vi "SwerveKinematics.vi"(8 "Rotation Center Choice":T1(ring), 9 "Joystick Rotation":dbl(slide) scale=1.0..-1.0, 10 "Joystick Y":dbl(slide) scale=-1.0..1.0, 11 "Joystick X":dbl(slide) scale=1.0..-1.0) -> (0 "Module 3 Velocity (ul)":dbl(slide) scale=0.0..1.0 scale format="%.2f", 1 "Module 2 Velocity (ul)":dbl(slide) scale=0.0..1.0 scale format="%.2f", 2 "Module 1 Velocity (ul)":dbl(slide) scale=0.0..1.0 scale format="%.2f", 3 "Module 0 Velocity (ul)":dbl(slide) scale=0.0..1.0 scale format="%.2f", 4 "Module 2 Angle (deg)":dbl(knob) scale=180.0..-180.0 scale format="%#_6f", 5 "Module 1 Angle (deg)":dbl(knob) scale=180.0..-180.0 scale format="%#_6f", 6 "Module 3 Angle (deg)":dbl(knob) scale=180.0..-180.0 scale format="%#_6f", 7 "Module 0 Angle (deg)":dbl(knob) scale=180.0..-180.0 scale format="%#_6f")   [LabVIEW 2019]
doc: "Performs the kinematics for a rectangular four wheel swerve robot with a selectable center of rotation. Swerve module #0 is located in the front right corner and the modules increment in the counter-clockwise direction."
panel:
  out "Angle 3 (deg) Old":dbl
  out "Angle 2 (deg) Old":dbl
  out "Angle 1 (deg) Old":dbl
  out "Velocity 3 (ul) Old":dbl format="%.2f"
  out "Velocity 2 (ul) Old":dbl format="%.2f"
  out "Velocity 1 (ul) Old":dbl format="%.2f"
  out "Velocity 0 (ul) Old":dbl format="%.2f"
  out "Angle 0 (deg) Old":dbl
  out "Velocity 3 (ul)":dbl format="%.2f"
  out "Velocity 2 (ul)":dbl format="%.2f"
  out "Velocity 1 (ul)":dbl format="%.2f"
  out "Velocity 0 (ul)":dbl format="%.2f"
  out "Angle 3 (deg) New":dbl
  out "Angle 2 (deg) New":dbl
  out "Angle 1 (deg) New":dbl
  out "Angle 0 (deg) New":dbl
  in  "Robot Width (in)":dbl=25.0
  in  "Robot Length (in)":dbl=25.0
  # "\"Front\" of Robot"
  # "M1"
  # "M0"
  # "Left Thumbstick"
  # "Right Thumbstick"
  # "X"
  # "Y"
  # "(0,0)"
  # "+CCW"
  # "M2"
  # "M3"
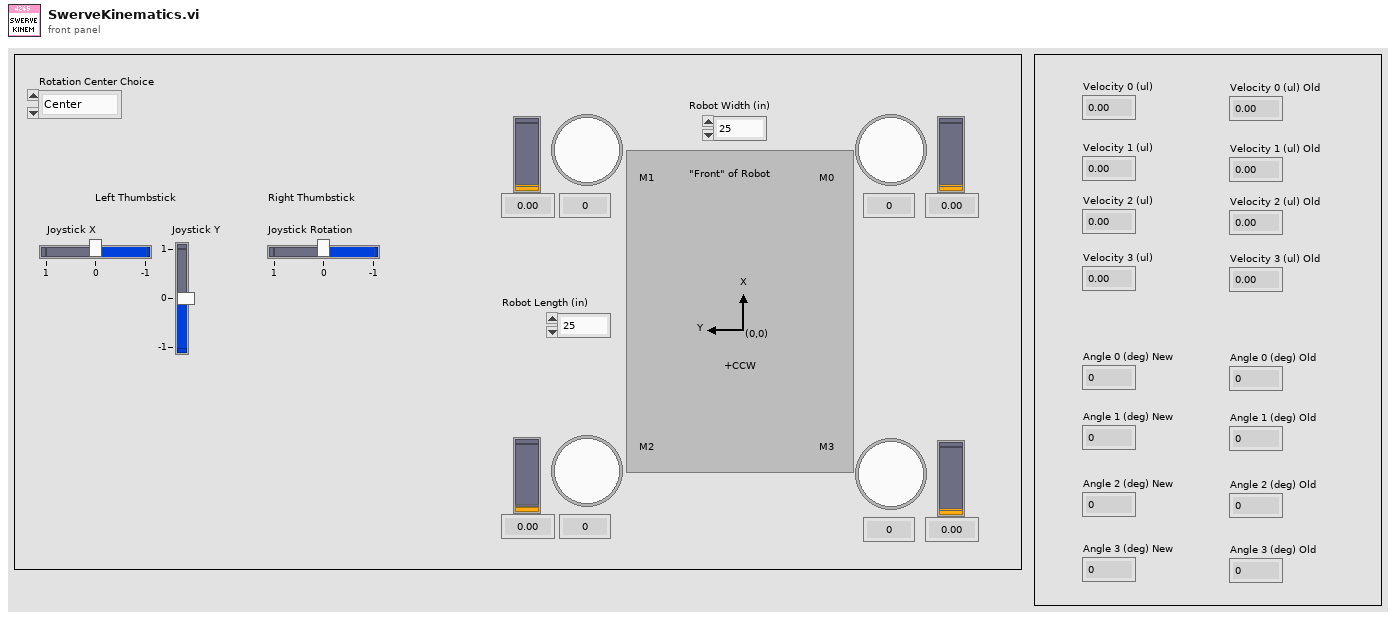
[diagram p1: front panel]
types:
  T1 = enum16{"Center", "Module 0", "Module 1", "Module 2", "Module 3"}
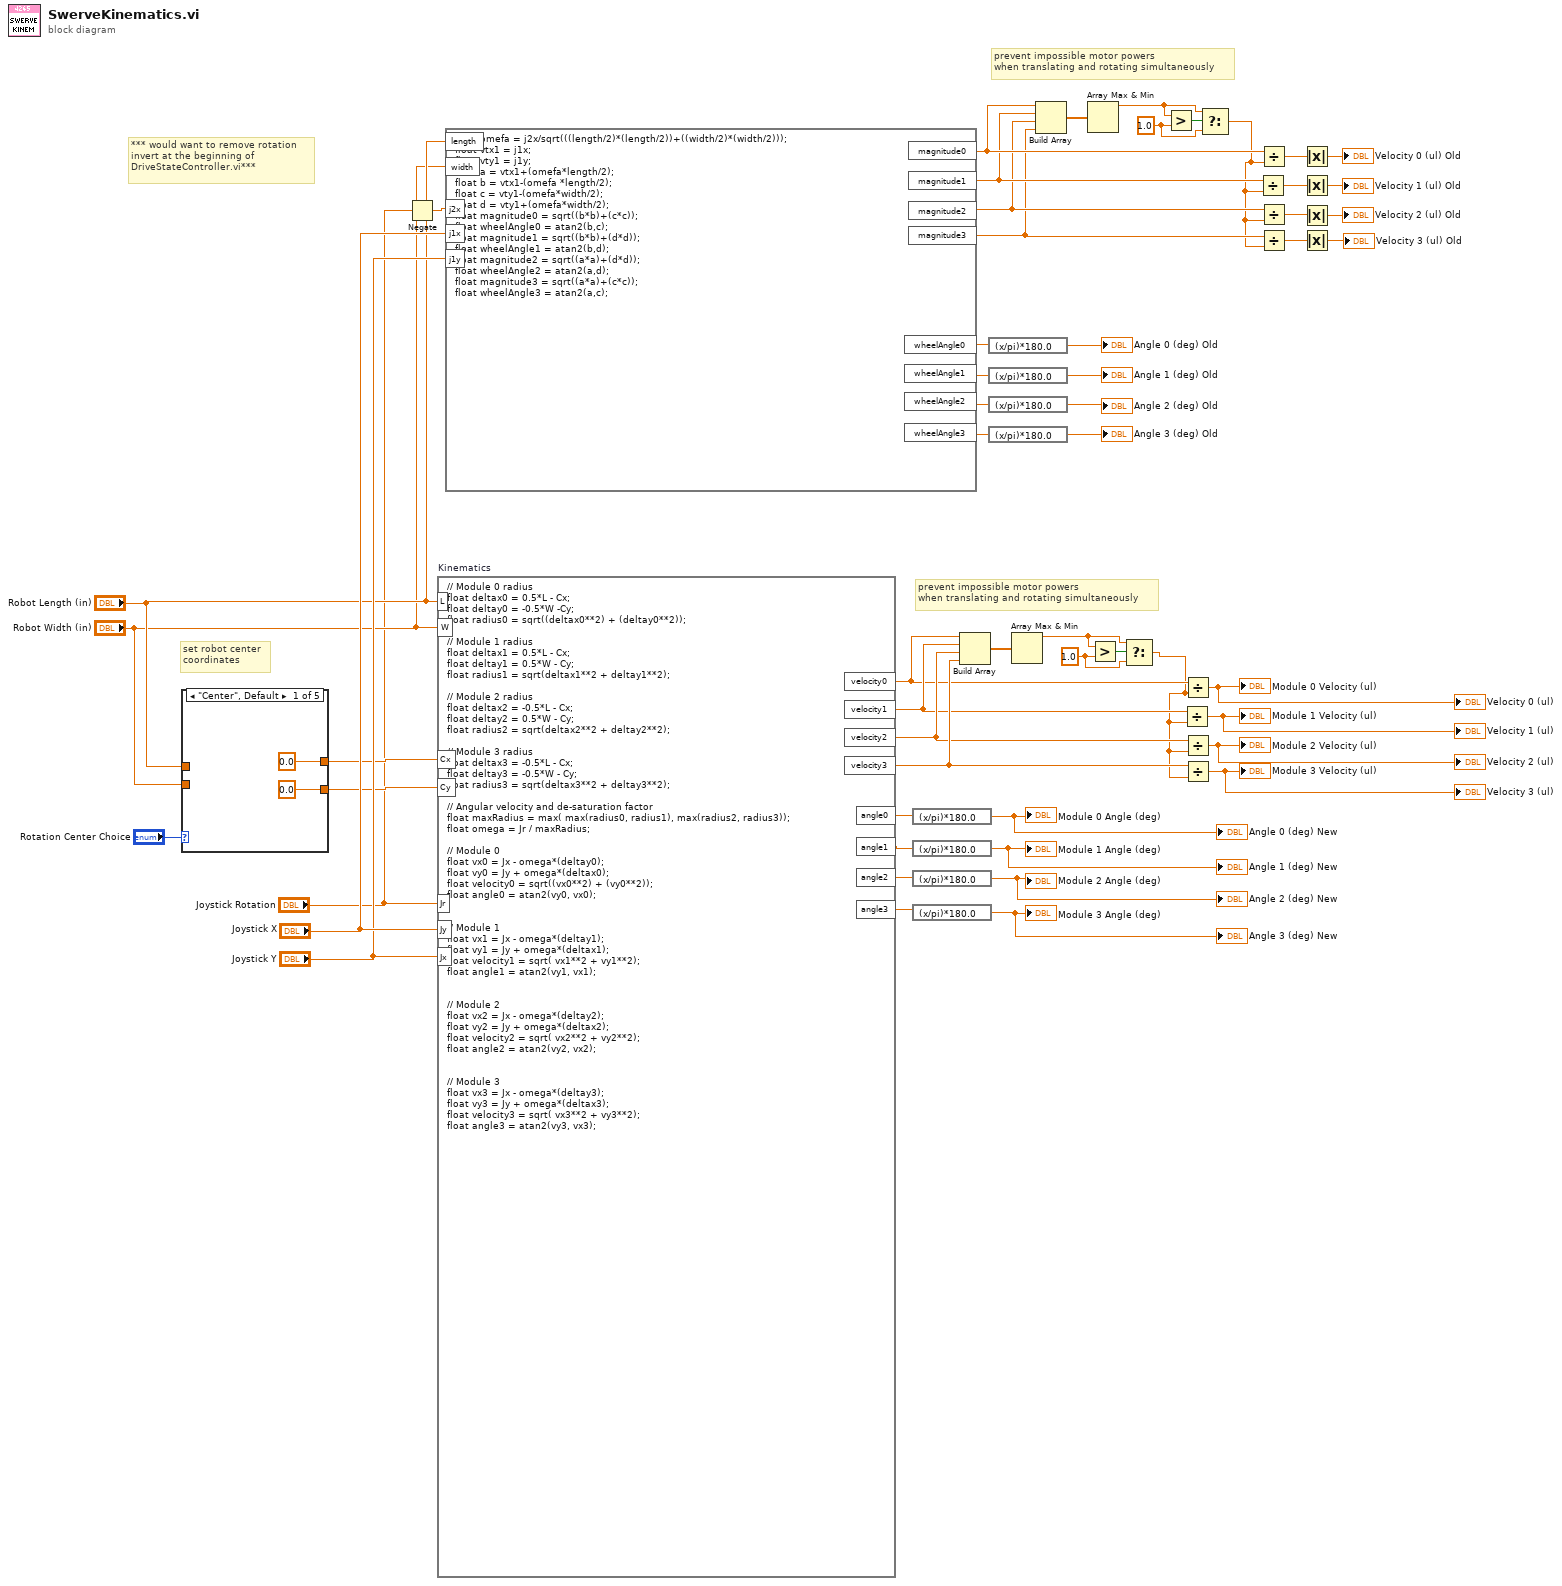
[diagram p0: block diagram]
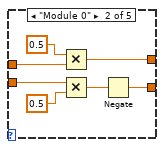
[diagram p2: hidden frame]
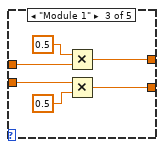
[diagram p3: hidden frame]
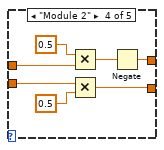
[diagram p4: hidden frame]
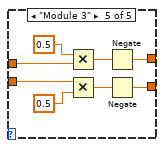
[diagram p5: hidden frame]
diagram:
  w25 = 1.0 ("y")
  w54 = 1.0 ("y")
  # "prevent impossible motor powers\nwhen translating and rotating simultaneously"
  # "set robot center \ncoordinates"
  # "*** would want to remove rotation\ninvert at the beginning of\nDriveStateController.vi***"
  # "prevent impossible motor powers\nwhen translating and rotating simultaneously"
  n1 = case shown="\"Center\", Default" "Rotation Center Choice" {
    tunnel: [0.0 w63 w66 w72 w79] -> w35
    tunnel: [0.0 w58 w65 w71 w78] -> w34
    tunnel: "Robot Length (in)" -> [_ w64 w68 w75 w83]
    tunnel: "Robot Width (in)" -> [_ w61 w67 w74 w82]
    frame "Center", Default {
    }
    frame "Module 0" {
      n2 = Multiply(x=0.5, y=w64) -> (x*y=w63:dbl)
      n3 = Multiply(x=w61, y=0.5) -> (x*y=w60:dbl)
      n4 = Negate(x=w60) -> (-x=w58:dbl)
    }
    frame "Module 1" {
      n5 = Multiply(x=0.5, y=w68) -> (x*y=w66:dbl)
      n6 = Multiply(x=w67, y=0.5) -> (x*y=w65:dbl)
    }
    frame "Module 2" {
      n7 = Multiply(x=0.5, y=w75) -> (x*y=w73:dbl)
      n8 = Multiply(x=w74, y=0.5) -> (x*y=w71:dbl)
      n9 = Negate(x=w73) -> (-x=w72:dbl)
    }
    frame "Module 3" {
      n10 = Multiply(x=0.5, y=w83) -> (x*y=w81:dbl)
      n11 = Multiply(x=w82, y=0.5) -> (x*y=w80:dbl)
      n12 = Negate(x=w81) -> (-x=w79:dbl)
      n13 = Negate(x=w80) -> (-x=w78:dbl)
    }
  }
  n14 = Negate(x="Joystick Rotation") -> (-x=w31:dbl)
  n15 = formula code="// Module 0 radius\nfloat deltax0 = 0.5*L - Cx;\nfloat deltay0 = -0.5*W -Cy; \nfloat radius0 = sqrt((deltax0**2) + (deltay0**2));\n\n// Module 1 radius\nfloat deltax1 = 0.5*L - Cx;\nfloat deltay1 = 0.5*W - Cy;\nfloat radius1 = sqrt(deltax1**2 + deltay1**2);\n\n// Module 2 radius\nfloat deltax2 = -0.5*L - Cx;\nfloat deltay2 = 0.5*W - Cy;\nfloat radius2 = sqrt(deltax2**2 + deltay2**2);\n\n// Module 3 radius\nfloat deltax3 = -0.5*L - Cx;\nfloat deltay3 = -0.5*W - Cy;\nfloat radius3 = sqrt(deltax3**2 + deltay3**2);\n\n// Angular velocity and de-saturation factor\nfloat maxRadius = max( max(radius0, radius1), max(radius2, radius3));\nfloat omega = Jr / maxRadius;\n\n// Module 0\nfloat vx0 = Jx - omega*(deltay0);\nfloat vy0 = Jy + omega*(deltax0);\nfloat velocity0 = sqrt((vx0**2) + (vy0**2));\nfloat angle0 = atan2(vy0, vx0);\n\n\n// Module 1\nfloat vx1 = Jx - omega*(deltay1);\nfloat vy1 = Jy + omega*(deltax1);\nfloat velocity1 = sqrt( vx1**2 + vy1**2);\nfloat angle1 = atan2(vy1, vx1);\n\n\n// Module 2\nfloat vx2 = Jx - omega*(deltay2);\nfloat vy2 = Jy + omega*(deltax2);\nfloat velocity2 = sqrt( vx2**2 + vy2**2);\nfloat angle2 = atan2(vy2, vx2);\n\n\n// Module 3\nfloat vx3 = Jx - omega*(deltay3);\nfloat vy3 = Jy + omega*(deltax3);\nfloat velocity3 = sqrt( vx3**2 + vy3**2);\nfloat angle3 = atan2(vy3, vx3);" "Kinematics"("L"="Robot Length (in)", "W"="Robot Width (in)", "Cx"=w35, "Cy"=w34, "Jr"="Joystick Rotation", "Jx"="Joystick Y", "Jy"="Joystick X") -> ("velocity0"=w19:dbl, "angle0"=w37:dbl, "angle1"=w29:dbl, "angle2"=w28:dbl, "angle3"=w27:dbl, "velocity1"=w20:dbl, "velocity2"=w21:dbl, "velocity3"=w22:dbl)
  n16 = formula code="float omefa = j2x/sqrt(((length/2)*(length/2))+((width/2)*(width/2)));\nfloat vtx1 = j1x;\nfloat vty1 = j1y;\nfloat a = vtx1+(omefa*length/2);\nfloat b = vtx1-(omefa *length/2);\nfloat c = vty1-(omefa*width/2);\nfloat d = vty1+(omefa*width/2);\nfloat magnitude0 = sqrt((b*b)+(c*c));\nfloat wheelAngle0 = atan2(b,c);\nfloat magnitude1 = sqrt((b*b)+(d*d));\nfloat wheelAngle1 = atan2(b,d);\nfloat magnitude2 = sqrt((a*a)+(d*d));\nfloat wheelAngle2 = atan2(a,d);\nfloat magnitude3 = sqrt((a*a)+(c*c));\nfloat wheelAngle3 = atan2(a,c);"("length"="Robot Length (in)", "width"="Robot Width (in)", "j2x"=w31, "j1y"="Joystick Y", "j1x"="Joystick X") -> ("wheelAngle0"=w45:dbl, "magnitude0"=w43:dbl, "magnitude1"=w42:dbl, "magnitude2"=w41:dbl, "magnitude3"=w40:dbl, "wheelAngle1"=w46:dbl, "wheelAngle2"=w47:dbl, "wheelAngle3"=w48:dbl)
  n17 = expression code="(x/pi)*180.0" ("radians to degrees")(w37) -> (→"Angle 0 (deg) New" →"Module 0 Angle (deg)":dbl)
  n18 = expression code="(x/pi)*180.0" ("radians to degrees")(w29) -> (→"Angle 1 (deg) New" →"Module 1 Angle (deg)":dbl)
  n19 = expression code="(x/pi)*180.0" ("radians to degrees")(w28) -> (→"Angle 2 (deg) New" →"Module 2 Angle (deg)":dbl)
  n20 = expression code="(x/pi)*180.0" ("radians to degrees")(w27) -> (→"Angle 3 (deg) New" →"Module 3 Angle (deg)":dbl)
  n21 = Build Array(w19, w20, w21, w22) -> (w23:dbl[])
  n22 = expression code="(x/pi)*180.0" ("radians to degrees")(w45) -> (→"Angle 0 (deg) Old":dbl)
  n23 = expression code="(x/pi)*180.0" ("radians to degrees")(w46) -> (→"Angle 1 (deg) Old":dbl)
  n24 = expression code="(x/pi)*180.0" ("radians to degrees")(w47) -> (→"Angle 2 (deg) Old":dbl)
  n25 = expression code="(x/pi)*180.0" ("radians to degrees")(w48) -> (→"Angle 3 (deg) Old":dbl)
  n26 = Array Max & Min(array=w23) -> (max value=w24:dbl)  [unwired: 3 out]
  n27 = Build Array(w43, w42, w41, w40) -> (w44:dbl[])
  n28 = Array Max & Min(array=w44) -> (max value=w53:dbl)  [unwired: 3 out]
  n29 = Greater?(x=w24, y=w25) -> (0:w26:bool)
  n30 = Select(t=w24, s=w26, f=w25) -> (s? t:f=w2:dbl)
  n31 = Greater?(x=w53, y=w54) -> (0:w55:bool)
  n32 = Divide(x=w20, y=w2) -> (x/y=→"Velocity 1 (ul)" →"Module 1 Velocity (ul)":dbl)
  n33 = Divide(x=w19, y=w2) -> (x/y=→"Velocity 0 (ul)" →"Module 0 Velocity (ul)":dbl)
  n34 = Divide(x=w21, y=w2) -> (x/y=→"Velocity 2 (ul)" →"Module 2 Velocity (ul)":dbl)
  n35 = Divide(x=w22, y=w2) -> (x/y=→"Velocity 3 (ul)" →"Module 3 Velocity (ul)":dbl)
  n36 = Select(t=w53, s=w55, f=w54) -> (s? t:f=w1:dbl)
  n37 = Divide(x=w42, y=w1) -> (x/y=w51:dbl)
  n38 = Divide(x=w43, y=w1) -> (x/y=w52:dbl)
  n39 = Divide(x=w41, y=w1) -> (x/y=w50:dbl)
  n40 = Divide(x=w40, y=w1) -> (x/y=w49:dbl)
  n41 = Absolute Value(x=w52) -> (abs(x)=→"Velocity 0 (ul) Old":dbl)
  n42 = Absolute Value(x=w51) -> (abs(x)=→"Velocity 1 (ul) Old":dbl)
  n43 = Absolute Value(x=w50) -> (abs(x)=→"Velocity 2 (ul) Old":dbl)
  n44 = Absolute Value(x=w49) -> (abs(x)=→"Velocity 3 (ul) Old":dbl)
